vi "Video Stuff v07.vi"() -> ()   [LabVIEW 2009]
uses:
  <vilib>/userDefined/High Color/IMAQdx.ctl
  <vilib>/vision/driver/NI_Vision_Acquisition_Software.lvlib
  <vilib>/vision/NI_Vision_Development_Module.lvlib
panel:
  out "Unit":T1
  out "X Resolution":i32
  out "Y Resolution":i32
  out "Image Type":T2 items=["Grayscale (U8)", "Grayscale (I16)", "Grayscale (SGL)", "Complex (CSG)", "RGB (U32)", "HSL (U32)", "RGB (U64)", "Grayscale (U16)"]
  in  "Numeric":i32
  in  "Calibration File Path":path
  in  "Save Calibration":bool
  in  "stop":bool
  out "Live Video":T3(plugin-control)
  in  "Video Modes":i32(listbox)
  in  "Camera Name":T4="cam0"
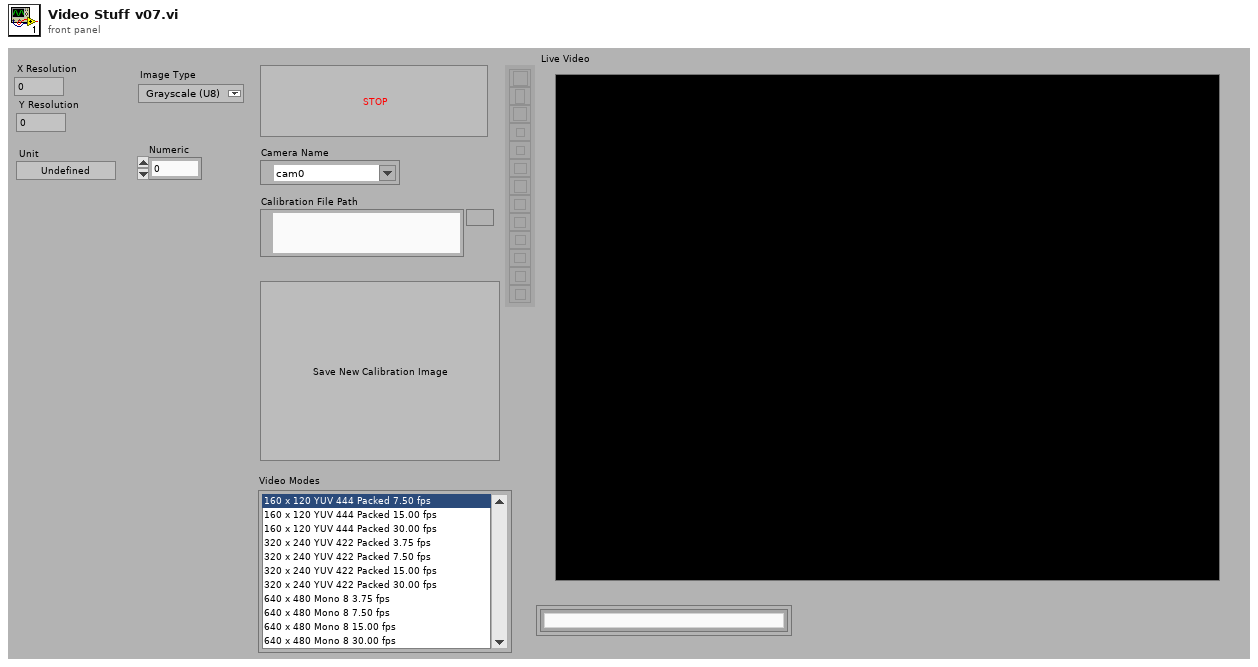
[diagram p1: front panel]
types:
  T1 = typedef "Image Unit" = enum32{"Undefined", "Angström", "Micrometer", "Millimeter", "Centimeter", "Meter", "Kilometer", "Microinch", "Inch", "Feet", "Nautical miles", "Standard miles", "Steps"}
  T2 = typedef "Image Type" = u32
  T3 = typedef "IMAQ Image.ctl" = refnum<image>
  T4 = typedef "IMAQdx.ctl" = refnum<k21>
  T5 = cluster{"X Step":sgl, "Y Step":sgl, "Unit":u32, "Threshold Range":cluster{"Lower value":sgl, "Upper value":sgl}}
  T6 = cluster{"Distortion":u32, "Corrected Image Scaling":u32, "Corrected Image Learn ROI":u32, "Learn Error Map?":bool, "Learn Correction Table?":bool}
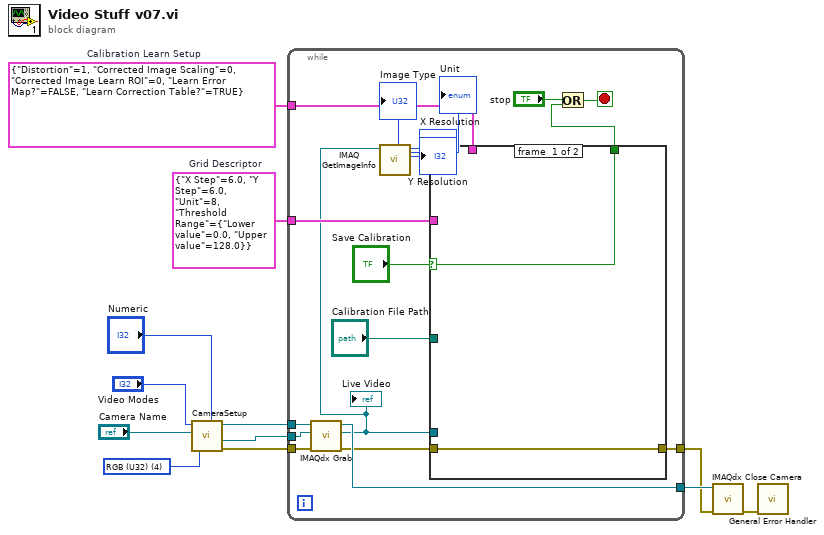
[diagram p0: block diagram]
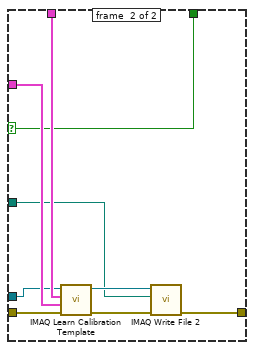
[diagram p2: hidden frame]
diagram:
  w7 = T2 4 items=["Grayscale (U8)", "Grayscale (I16)", "Grayscale (SGL)", "Complex (CSG)", "RGB (U32)", "HSL (U32)", "RGB (U64)", "Grayscale (U16)"] ("Image Type")
  w2 = T5 {"X Step"=6.0, "Y Step"=6.0, "Unit"=8, "Threshold Range"={"Lower value"=0.0, "Upper value"=128.0}}  # Grid Descriptor
  w3 = T6 {"Distortion"=1, "Corrected Image Scaling"=0, "Corrected Image Learn ROI"=0, "Learn Error Map?"=FALSE, "Learn Correction Table?"=TRUE}  # Calibration Learn Setup
  n1 = call "CameraSetup.vi"("Video Modes"="Video Modes", "Camera Name"="Camera Name", "Image Type"=w7, "Numeric"="Numeric") -> ("Session Out"=w10:T4, "New Image"=w9:T3, "error out"=w8:errorcluster)  [unwired: 2 in]
  n2 = while {
    tunnel: w10 -> [w30]
    tunnel: w9 -> [w29]
    tunnel: w8 -> [w28]
    tunnel: [w27] -> w5
    tunnel: [w24] -> w4
    tunnel: w3 -> [w22]
    tunnel: w2 -> [w21]
    stop <- w19 stop-if-true
    n3 = call <vilib>:"IMAQdx Grab.vi"("error in"=w28, "Image In"=w29, "Session In"=w30) -> ("error out"=w26:errorcluster, "Image Out"=w17:T3, "Session Out"=w27:T4)  [unwired: 1 in, 5 out]
    "Live Video" <- w17
    n4 = call "IMAQ GetImageInfo"("Image"=w17) -> ("Y Resolution"=→"Y Resolution":i32, "X Resolution"=→"X Resolution":i32, "Unit"=→"Unit":T1, "Image Type"=→"Image Type":T2)  [unwired: 3 in, 4 out]
    n5 = case shown="True" "Save Calibration" {
      selector: "Save Calibration" -> [w31 w33]
      tunnel: w17 -> [_ w38]
      tunnel: w26 -> [w32 w41]
      tunnel: [w32 w34] -> w24
      tunnel: "Calibration File Path" -> [_ w36]
      tunnel: w22 -> [_ w40]
      tunnel: w21 -> [_ w39]
      tunnel: [w31 w33] -> w18
      frame #0 {
      }
      frame #1 {
        n6 = call "IMAQ Learn Calibration Template"("error in (no error)"=w41, "Grid Descriptor"=w39, "Calibration Learn Setup"=w40, "Image"=w38) -> ("error out"=w35:errorcluster, "Calibrated Image"=w37:T3)  [unwired: 3 in, 3 out]
        n7 = call-poly "IMAQ Write File 2"("error in (no error)"=w35, "File Path"=w36, "Image"=w37) -> ("error out"=w34:errorcluster)  [unwired: 7 in, 1 out]
      }
    }
    n8 = Or(x="stop", y=w18) -> (x .or. y?=w19:bool)
  }
  n9 = call <vilib>:"IMAQdx Close Camera.vi"("error in"=w4, "Session In"=w5) -> ("error out"=w6:errorcluster)  [unwired: 9 out]
  n10 = call <vilib>:"General Error Handler.vi"("error in (no error)"=w6) -> ()  [unwired: 1 in, 14 out]
